vi "Task - Pressure & Flow - Original.vi"() -> ()   [LabVIEW 2013]
uses:
  <vilib>/Utility/error.llb/DialogType.ctl
  Global - Pressure & Flow.vi
panel:
  in  "MilliSec per Cycle":i32=250
  in  "#Cycles":i32=100000
  out "Temperature (K)":dbl=2.13410741378
  out "Output Pressure":dbl=33.964
  out "Vapor Pressure":T1(graph)={"Pressure value"=33.964, "Converted Output"=2.13410741378}
  out "Target Cavity Flow\n(SLM)":dbl(slide)=0.02 scale=0.0..100.0
  out "Separator Flow\n(SLM)":dbl(slide)=-0.0035 scale=0.0..100.0
  out "Target Cavity Flow\n(SLM)":dbl=0.02
  out "Separator Flow\n(SLM)":dbl=-0.0035
  out "Pressure (Torr)":dbl=34.2
  out "Pressure (Torr)":dbl=33.964
  in  "MKS 946 Low-res":refnum<visa-resource-name>="COM5"
  in  "MKS 670 Hi-res P":refnum<visa-resource-name>="COM6"
  in  "error in (no error)":errorcluster
  out "error out":errorcluster={"status"=FALSE, "code"=3003, "source"="Task1 completed OK at 100 cycles"}
  out "Time Stamp":timestamp=timestamp(3561144723.7158904 s since 1904-01-01)
  out "stop":bool=TRUE
  out "Heartbeat":bool
  out "Finished":bool=TRUE
  out "Cycle":i32=101
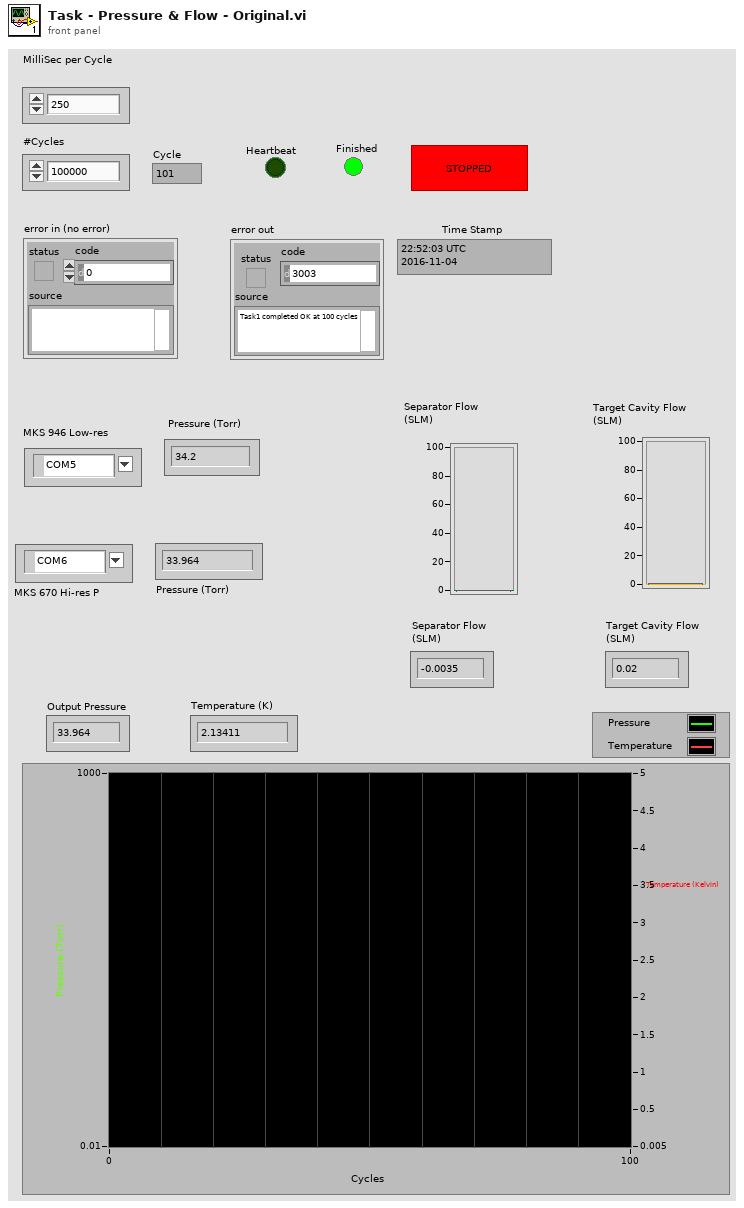
[diagram p1: front panel]
types:
  T1 = cluster{"Pressure value":dbl, "Converted Output":dbl}
  T2 = enum16{"MKS946 High Pressure Gauge", "MKS946 Separator Flow", "MKS946 Target Cavity Flow", "MKS670 Low Pressure Gauge"}
  T3 = typedef "DialogType.ctl" = u16
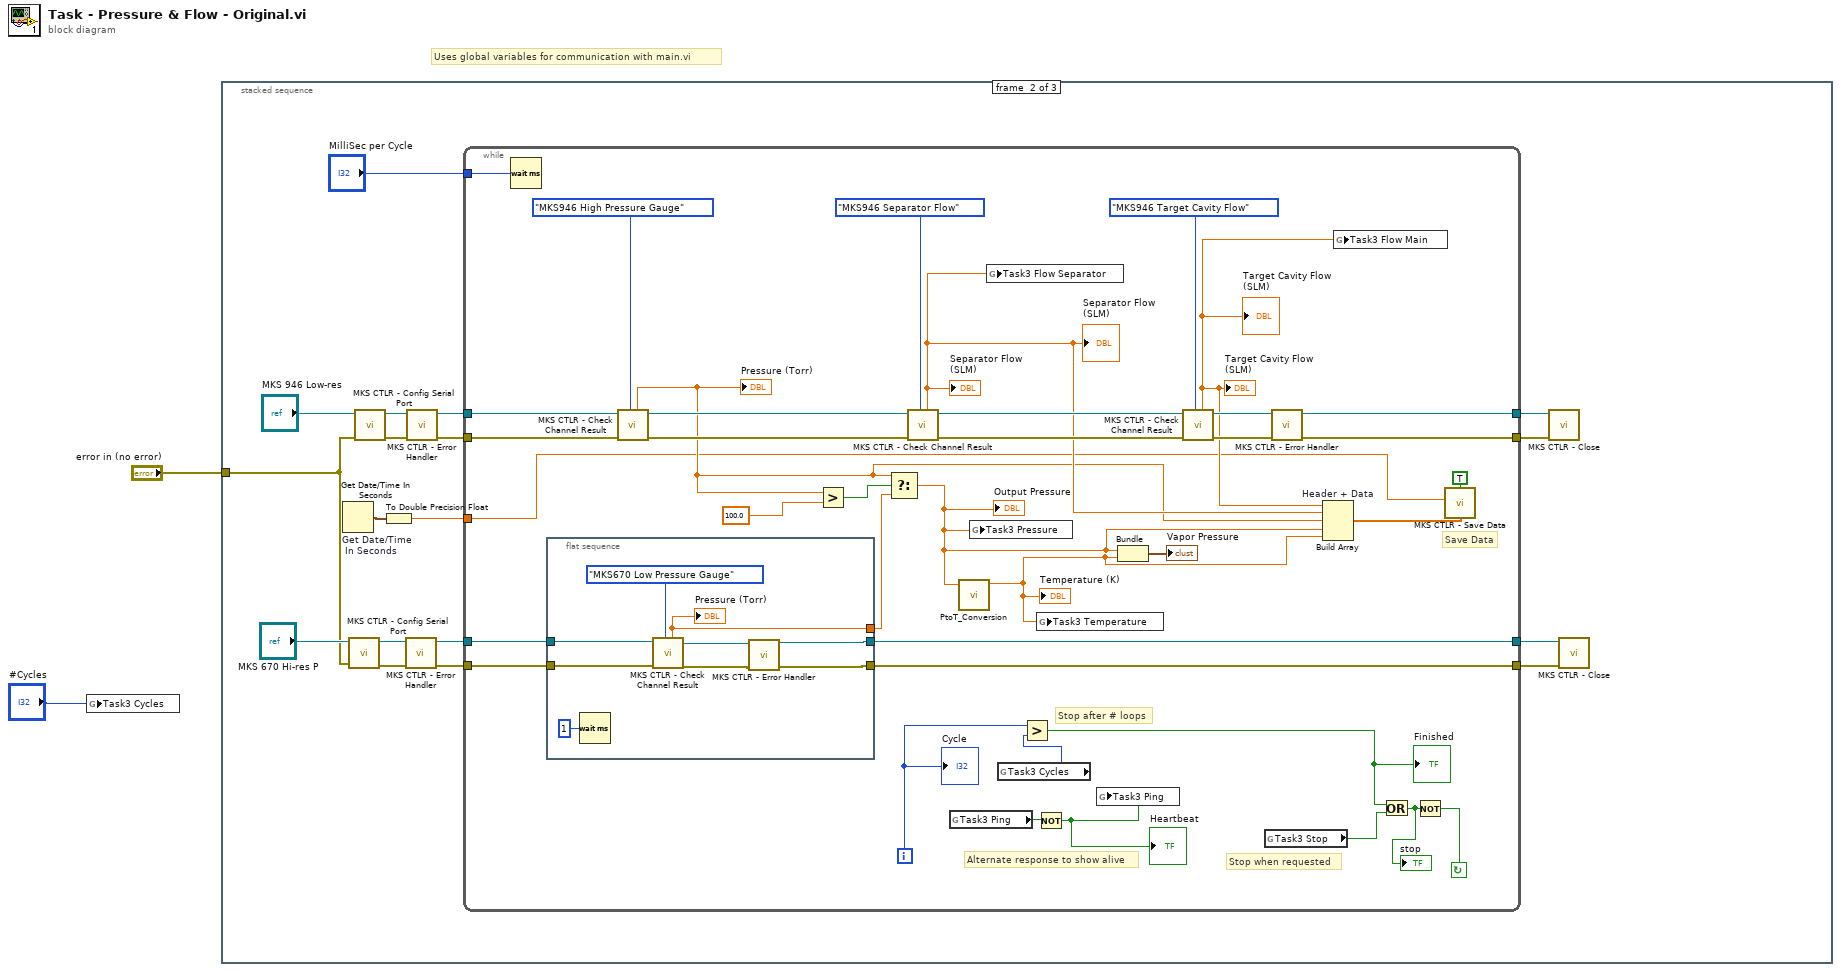
[diagram p0: block diagram]
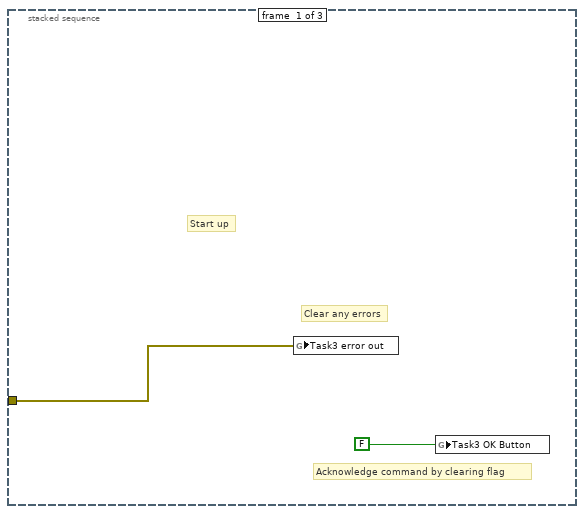
[diagram p2: hidden frame]
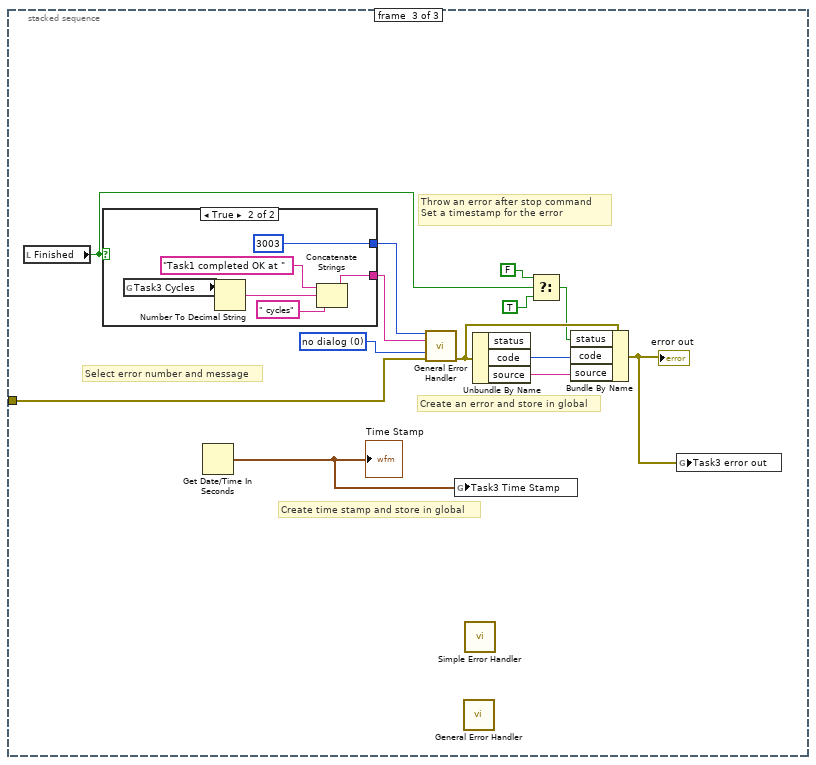
[diagram p3: hidden frame]
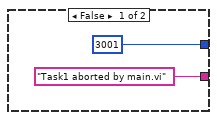
[diagram p4: hidden frame]
diagram:
  # "Uses global variables for communication with main.vi"
  n1 = global write "Global - Pressure & Flow.vi" "Task3 Cycles"("#Cycles") -> ()
  n2 = stacked-sequence {
    tunnel: "error in (no error)" -> [w4 w20 w81]
    frame #0 {
      # "Start up"
      # "Acknowledge command by clearing flag"
      # "Clear any errors"
      n3 = global write "Global - Pressure & Flow.vi" "Task3 error out"(w4) -> ()
      n4 = global write "Global - Pressure & Flow.vi" "Task3 OK Button"(FALSE) -> ()
    }
    frame #1 {
      n5 = Get Date/Time In Seconds "Get Date/Time\n In Seconds"() -> (seconds since 1Jan1904=w7:timestamp)
      n6 = call "MKS CTLR - Config Serial Port.vi"("Error In"=w20, "MKS ViiSA resource name in"="MKS 670 Hi-res P") -> ("Error Out"=w11:errorcluster, "VISA resource name out"=w12:refnum<visa-resource-name>)  [unwired: 8 in]
      n7 = call "MKS CTLR - Config Serial Port.vi"("Error In"=w20, "MKS ViiSA resource name in"="MKS 946 Low-res") -> ("Error Out"=w14:errorcluster, "VISA resource name out"=w13:refnum<visa-resource-name>)  [unwired: 8 in]
      n8 = To Double Precision Float(number=w7) -> (double precision float=w6:dbl)
      n9 = call "MKS CTLR - Error Handler.vi"("error in (no error)"=w11, "VISA resource name (IN)"=w12) -> ("error out"=w10:errorcluster, "VISA resource name (OUT)"=w9:refnum<visa-resource-name>)  [unwired: 8 in]
      n10 = call "MKS CTLR - Error Handler.vi"("error in (no error)"=w14, "VISA resource name (IN)"=w13) -> ("error out"=w15:errorcluster, "VISA resource name (OUT)"=w16:refnum<visa-resource-name>)  [unwired: 8 in]
      n11 = while {
        tunnel: w16 -> [w32]
        tunnel: w15 -> [w33]
        tunnel: w10 -> [w34]
        tunnel: [w37] -> w19
        tunnel: [w45] -> w18
        tunnel: [w44] -> w17
        tunnel: w9 -> [w35]
        tunnel: [w36] -> w5
        tunnel: "MilliSec per Cycle" -> [w31]
        tunnel: w6 -> [w23]
        i -> [w53]
        stop <- w60 continue-if-true
        # "Save Data"
        # "Stop after # loops"
        # "Alternate response to show alive"
        # "Stop when requested"
        n12 = Wait (ms)(milliseconds to wait=w31) -> ()  [unwired: 1 out]
        n13 = flat-sequence {
          tunnel: w35 -> [w69]
          tunnel: w34 -> [w68]
          tunnel: [w62] -> w44
          tunnel: [w61] -> w45
          tunnel: [w65] -> w41
          frame #0 {
            n14 = Wait (ms)(milliseconds to wait=u32 1) -> ()  [unwired: 1 out]
            n15 = call "MKS CTLR - Check Channel Result.vi"("Channel"=T2."MKS670 Low Pressure Gauge", "error in (no error)"=w68, "VISA resource name (IN)"=w69) -> ("error out"=w63:errorcluster, "VISA resource name (OUT)"=w64:refnum<visa-resource-name>, "Pressure value"=w65:dbl)  [unwired: 5 in, 1 out]
            "Pressure (Torr)" <- w65
            n16 = call "MKS CTLR - Error Handler.vi"("error in (no error)"=w63, "VISA resource name (IN)"=w64) -> ("error out"=w62:errorcluster, "VISA resource name (OUT)"=w61:refnum<visa-resource-name>)  [unwired: 8 in]
          }
        }
        n17 = call "MKS CTLR - Check Channel Result.vi"("Channel"=T2."MKS946 High Pressure Gauge", "error in (no error)"=w33, "VISA resource name (IN)"=w32) -> ("error out"=w49:errorcluster, "VISA resource name (OUT)"=w50:refnum<visa-resource-name>, "Pressure value"=w26:dbl)  [unwired: 5 in, 1 out]
        "Pressure (Torr)" <- w26
        n18 = Greater?(x=w26, y=100.0) -> (0:w42:bool)
        n19 = Select(t=w26, s=w42, f=w41) -> (s? t:f=w25:dbl)
        "Output Pressure" <- w25
        n20 = call "MKS CTLR - Check Channel Result.vi"("Channel"=T2."MKS946 Separator Flow", "error in (no error)"=w49, "VISA resource name (IN)"=w50) -> ("error out"=w46:errorcluster, "VISA resource name (OUT)"=w47:refnum<visa-resource-name>, "Pressure value"=w29:dbl)  [unwired: 5 in, 1 out]
        "Separator Flow\n(SLM)" <- w29
        "Separator Flow\n(SLM)" <- w29
        n21 = global read "Global - Pressure & Flow.vi" "Task3 Ping"() -> (w59:bool)
        n22 = call "PtoT_Conversion.vi"("A"=w25) -> ("Converted Output"=w27:dbl)  [unwired: 9 in, 1 out]
        "Temperature (K)" <- w27
        n23 = global write "Global - Pressure & Flow.vi" "Task3 Pressure"(w25) -> ()
        n24 = global write "Global - Pressure & Flow.vi" "Task3 Flow Separator"(w29) -> ()
        n25 = global read "Global - Pressure & Flow.vi" "Task3 Cycles"() -> (w54:i32)
        n26 = Greater?(x=w53, y=w54) -> (0:w56:bool)
        "Finished" <- w56
        n27 = Not(x=w59) -> (.not. x?=w58:bool)
        "Heartbeat" <- w58
        n28 = global write "Global - Pressure & Flow.vi" "Task3 Temperature"(w27) -> ()
        n29 = global write "Global - Pressure & Flow.vi" "Task3 Ping"(w58) -> ()
        n30 = Bundle("Pressure value"=w25, "Converted Output"=w27) -> (→"Vapor Pressure":T1)  [unwired: 1 in]
        n31 = call "MKS CTLR - Check Channel Result.vi"("Channel"=T2."MKS946 Target Cavity Flow", "error in (no error)"=w46, "VISA resource name (IN)"=w47) -> ("error out"=w38:errorcluster, "VISA resource name (OUT)"=w39:refnum<visa-resource-name>, "Pressure value"=w30:dbl)  [unwired: 5 in, 1 out]
        "Target Cavity Flow\n(SLM)" <- w30
        "Target Cavity Flow\n(SLM)" <- w30
        n32 = global read "Global - Pressure & Flow.vi" "Task3 Stop"() -> (w57:bool)
        n33 = call "MKS CTLR - Error Handler.vi"("error in (no error)"=w38, "VISA resource name (IN)"=w39) -> ("error out"=w36:errorcluster, "VISA resource name (OUT)"=w37:refnum<visa-resource-name>)  [unwired: 8 in]
        n34 = Build Array "Header + Data"(w30, w29, w26, w25, w27) -> (w28:dbl[])
        n35 = global write "Global - Pressure & Flow.vi" "Task3 Flow Main"(w30) -> ()
        n36 = Or(x=w56, y=w57) -> (x .or. y?=w55:bool)
        "stop" <- w55
        n37 = Not(x=w55) -> (.not. x?=w60:bool)
        n38 = call "MKS CTLR - Save Data.vi"("Array"=w28, "Save Data to File"=TRUE, "Ext time (sec)"=w23) -> ()  [unwired: 1 out]
        "Cycle" <- w53
      }
      n39 = call "MKS CTLR - Close.vi"("error in (no error)"=w5, "VISA resource name (IN)"=w19) -> ()  [unwired: 9 in, 1 out]
      n40 = call "MKS CTLR - Close.vi"("error in (no error)"=w17, "VISA resource name (IN)"=w18) -> ()  [unwired: 9 in, 1 out]
    }
    frame #2 {
      w82 = T3 0 items=["no dialog", "OK message", "continue or stop message", "OK message + warnings", "continue/stop + warnings"] ("type of dialog (OK msg:1)")
      # "Create time stamp and store in global"
      # "Select error number and message"
      # "Throw an error after stop command\nSet a timestamp for the error"
      # "Create an error and store in global"
      n41 = local read "Finished"() -> (w77:bool)
      n42 = case shown="True" w77 {
        tunnel: [3001 ("[error code] (0)") 3003 ("[error code] (0)")] -> w78
        tunnel: ["Task1 aborted by main.vi" ("[error source] (\" \")") w85] -> w79
        frame False {
        }
        frame True {
          n43 = global read "Global - Pressure & Flow.vi" "Task3 Cycles"() -> (w89:i32)
          n44 = Number To Decimal String(number=w89) -> (decimal integer string=w87:string)  [unwired: 1 in]
          n45 = Concatenate Strings("Task1 completed OK at " ("[error source] (\" \")"), w87, " cycles") -> (w85:string)
        }
      }
      n46 = Get Date/Time In Seconds() -> (seconds since 1Jan1904=w80:timestamp)
      "Time Stamp" <- w80
      n47 = call <vilib>:"General Error Handler.vi"("[error code] (0)"=w78, "[error source] (\" \")"=w79, "type of dialog (OK msg:1)"=w82, "error in (no error)"=w81) -> ("error out"=w72:errorcluster)  [unwired: 7 in, 4 out]
      n48 = global write "Global - Pressure & Flow.vi" "Task3 Time Stamp"(w80) -> ()
      n49 = call <vilib>:"General Error Handler.vi"() -> ()  [unwired: 11 in, 5 out]
      n50 = call <vilib>:"Simple Error Handler.vi"() -> ()  [unwired: 5 in, 5 out]
      n51 = Unbundle By Name(w72) -> ("code"=w74:i32, "source"=w73:string)  [unwired: 1 out]
      n52 = Select(t=FALSE, s=w77, f=TRUE) -> (s? t:f=w70:bool)
      n53 = Bundle By Name(cluster=w72, "status"=w70, "code"=w74, "source"=w73) -> (w71:errorcluster)
      "error out" <- w71
      n54 = global write "Global - Pressure & Flow.vi" "Task3 error out"(w71) -> ()
    }
  }
